vi "Test MxThV10 v2.vi"() -> ()   [LabVIEW 2017]
uses:
  <vilib>/Platform/TimedLoop/XDataNode/timing_clust.ctl
  <vilib>/Platform/TimedLoop/XDataNode/nitl_modes.ctl
  <vilib>/Platform/TimedLoop/XDataNode/wakeup.ctl
  <vilib>/platform/TimedLoop/XDataNode/XDataNode.xnode
  <vilib>/Platform/TimedLoop/XDataNode/XDNodeRunTimeDep.lvlib
panel:
  out "data file":string
  in  "com port":refnum<visa-resource-name>
  out "ID":dbl
  in  "Channel":string
  out "tdms file out":refnum<k34>
  in  "Stop Button":bool
  out "CYCLES":dbl
  out "cycle":bool
  out "error":bool
  out "T4":dbl
  out "T3":dbl
  out "T2":dbl
  out "T1":dbl
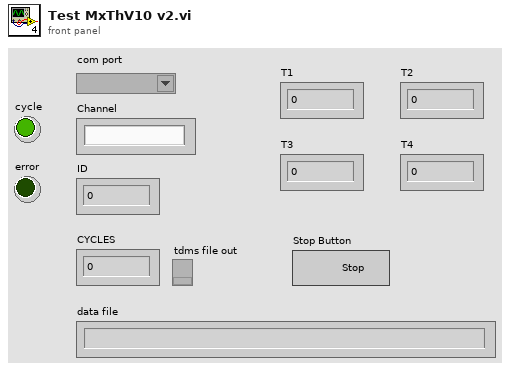
[diagram p1: front panel]
types:
  T1 = enum16{"open", "open or create", "create or replace", "create", "open (read-only)"}
  T2 = typedef "XDNodeRunTimeDep.lvlib/timing_clust.ctl" = cluster{"Expected End [f-1]":u64, "Actual End [f-1]":u64, "Finished Late? [f-1]":bool, "Expected End [i-1]":u64, "Actual End [i-1]":u64, "Finished Late? [i-1]":bool, "Expected Start [i]":u64, "Actual Start [i]":u64, "Expected Start [f]":u64, "Actual Start [f]":u64, "Source Name":string, "Structure Name":string, "Period":i64, "Deadline":i64, "Offset":i64, "Start":i64, "Priority":i32, "Timeout":i32, "Mode":T3, "Wakeup Reason":T4, "Error":errorcluster, "Source Type":string, "Secondary Source Type":string, "Global End Time":u64, "Global Start Time":u64, "Frame Duration":u64, "Iteration Duration":u64, "Assigned CPU":i32, "I/O Scan Engine Mode":u32}
  T3 = typedef "XDNodeRunTimeDep.lvlib/nitl_modes.ctl" = enum32{"No Change", "Process missed periods, maintain original phase", "Discard missed periods, maintain original phase", "Process missed periods, ignore original phase", "Discard missed periods, ignore original phase"}
  T4 = typedef "XDNodeRunTimeDep.lvlib/wakeup.ctl" = enum32{"Normal", "Aborted", "Asynchronous wakeup", "Timing source error", "Timed loop error", "Timeout"}
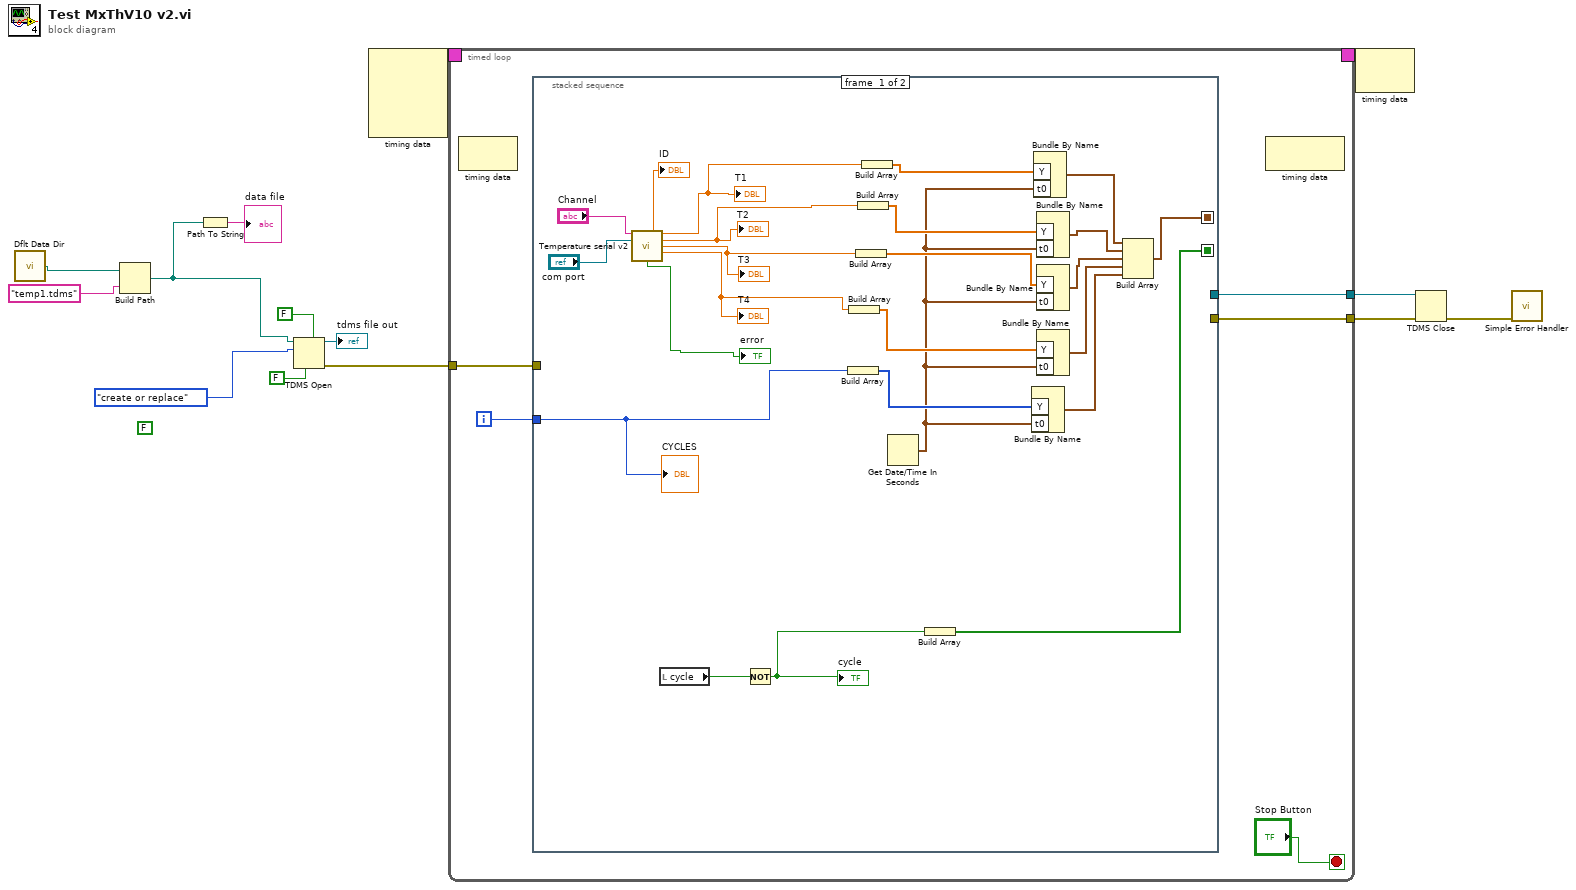
[diagram p0: block diagram]
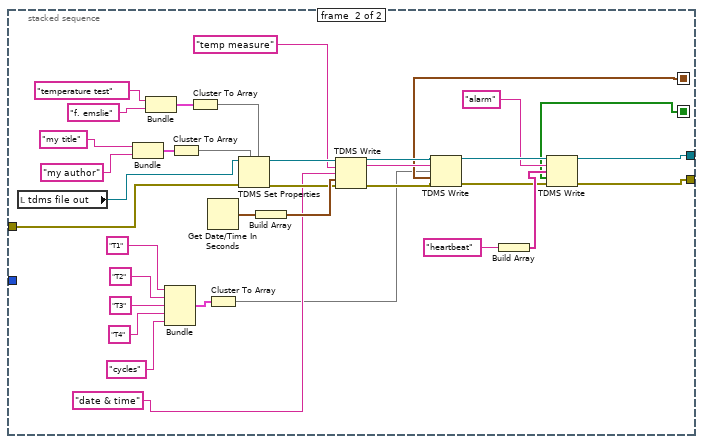
[diagram p2: hidden frame]
diagram:
  (unwired) FALSE
  n1 = call <vilib>:"Dflt Data Dir.vi"() -> ("App:Default Data Directory"=w1:path)
  n2 = Build Path(base path=w1, name or relative path="temp1.tdms") -> (appended path=w2:path)
  n3 = Path To String(path=w2) -> (string=→"data file":string)
  n4 = TDMS Open(5:FALSE ("create index file? (T)"), 6:FALSE ("disable buffering? (T)"), 10:T1."create or replace" ("operation (0:open)"), 11:w2) -> (0:w10:errorcluster, 3:→"tdms file out":refnum<k34>)  [unwired: 3 in]
  n5 = node-c288() -> (w14:T2)  [unwired: 4 in]
  n6 = timed-loop {
    timing: w14 -> [_]
    timing-out: [_] -> w13
    tunnel: w10 -> [w17]
    tunnel: [w16] -> w9
    tunnel: [w15] -> w8
    i -> [w19]
    stop <- "Stop Button" stop-if-true
    n7 = node-c288() -> ()  [unwired: 1 in, 1 out]
    n8 = stacked-sequence {
      seq-local: [w28 _] -> [_ w54]
      seq-local: [w23 _] -> [_ w49]
      tunnel: w19 -> [w41 _]
      tunnel: w17 -> [_ w63]
      tunnel: [_ w47] -> w16
      tunnel: [_ w46] -> w15
      frame #0 {
        n9 = call "Temperature serial v2.vi"("Command String"="Channel", "com port"="com port") -> ("ID"=→"ID":dbl, "T1"=w39:dbl, "T2"=w38:dbl, "T3"=w37:dbl, "T4"=w36:dbl, "error"=→"error":bool)  [unwired: 7 in, 1 out]
        "T2" <- w38
        "T4" <- w36
        "T1" <- w39
        "T3" <- w37
        n10 = local read "cycle"() -> (w43:bool)
        n11 = Not(x=w43) -> (.not. x?=w40:bool)
        "cycle" <- w40
        n12 = Build Array(w41) -> (w31:i32[])
        n13 = Build Array(w36) -> (w32:dbl[])
        n14 = Build Array(w37) -> (w33:dbl[])
        n15 = Build Array(w38) -> (w34:dbl[])
        n16 = Build Array(w39) -> (w35:dbl[])
        n17 = Get Date/Time In Seconds() -> (seconds since 1Jan1904=w29:timestamp)
        n18 = Build Array(w40) -> (w23:bool[])
        n19 = Bundle By Name("Y"=w31, "t0"=w29) -> (w24:waveform(i32))  [unwired: 1 in]
        n20 = Bundle By Name("Y"=w35, "t0"=w29) -> (w30:waveform(dbl))  [unwired: 1 in]
        n21 = Bundle By Name("Y"=w34, "t0"=w29) -> (w27:waveform(dbl))  [unwired: 1 in]
        n22 = Bundle By Name("Y"=w33, "t0"=w29) -> (w26:waveform(dbl))  [unwired: 1 in]
        n23 = Bundle By Name("Y"=w32, "t0"=w29) -> (w25:waveform(dbl))  [unwired: 1 in]
        n24 = Build Array(w30, w27, w26, w25, w24) -> (w28:waveform(dbl)[])
        "CYCLES" <- w41
      }
      frame #1 {
        n25 = local read "tdms file out"() -> (w45:refnum<k34>)
        n26 = Bundle("my title", "my author") -> (w66:cluster{string, string})  [unwired: 1 in]
        n27 = Bundle("temperature test", "f. emslie") -> (w69:cluster{string, string})  [unwired: 1 in]
        n28 = Bundle("T1", "T2", "T3", "T4", "cycles") -> (w74:cluster{string, string, string, string, string})  [unwired: 1 in]
        n29 = Cluster To Array(cluster=w66) -> (array=w67:string[])
        n30 = Cluster To Array(cluster=w69) -> (array=w65:string[])
        n31 = Get Date/Time In Seconds() -> (seconds since 1Jan1904=w72:timestamp)
        n32 = Cluster To Array(cluster=w74) -> (array=w44:string[])
        n33 = TDMS Set Properties(5:w65, 7:w67, 8:w63, 11:w45) -> (0:w61:errorcluster, 3:w60:refnum<k34>)  [unwired: 2 in, 2 out]
        n34 = Build Array(w72) -> (w62:timestamp[])
        n35 = TDMS Write(0:w60, 5:"temp measure", 7:"date & time", 9:w62, 11:w61) -> (4:w56:refnum<k34>, 6:w55:string, 15:w57:errorcluster)  [unwired: 1 in, 1 out]
        n36 = TDMS Write(0:w56, 5:w55, 7:w44, 9:w54, 11:w57) -> (4:w53:refnum<k34>, 15:w48:errorcluster)  [unwired: 1 in, 2 out]
        n37 = Build Array("heartbeat") -> (w50:string[])
        n38 = TDMS Write(0:w53, 5:"alarm", 7:w50, 9:w49, 11:w48) -> (4:w47:refnum<k34>, 15:w46:errorcluster)  [unwired: 1 in, 2 out]
      }
    }
    n39 = node-c288() -> ()  [unwired: 1 in, 1 out]
  }
  n40 = node-c288(w13) -> ()  [unwired: 1 out]
  n41 = TDMS Close(8:w8, 11:w9) -> (0:w7:errorcluster)  [unwired: 1 out]
  n42 = call <vilib>:"Simple Error Handler.vi"("error in (no error)"=w7) -> ()  [unwired: 4 in, 5 out]
